vi "st_independent seeds.vi"(9 "number of seeds":i32=2, 10 "seed":i32=-1) -> (2 "independent seeds":i32[](array[numeric]))   [LabVIEW 2014, in "NI_Gmath.lvlib"]
uses:
  NI_Gmath.lvlib
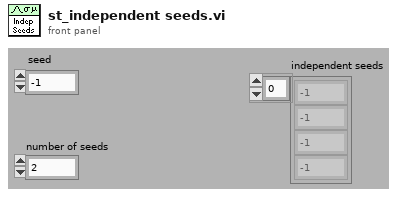
[diagram p1: front panel]
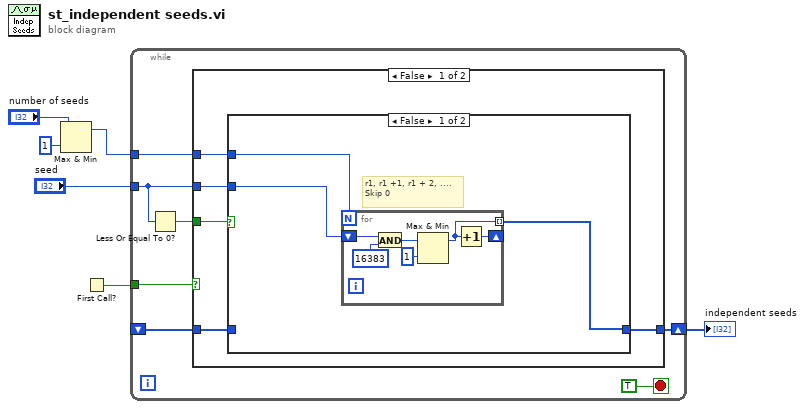
[diagram p0: block diagram]
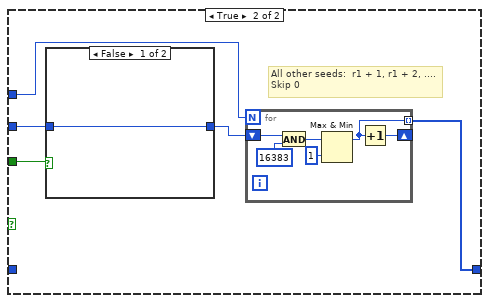
[diagram p3: hidden frame]
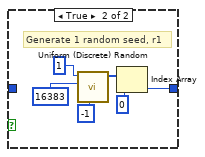
[diagram p4: hidden frame]
diagram:
  n1 = Max & Min(x="number of seeds", y=1) -> (max(x,y)=w2:i32)  [unwired: 1 out]
  n2 = First Call?() -> (First Call?: T/F=w5:bool)
  n3 = while {
    tunnel: w2 -> [w13]
    tunnel: "seed" -> [w11]
    shift-right: [w7] -> w1
    shift-left: _ -> [w12]
    tunnel: w5 -> [w9]
    stop <- TRUE stop-if-true
    n4 = Less Or Equal To 0?(x=w11) -> (x <= 0?=w10:bool)
    n5 = case shown="False" w9 {
      tunnel: w13 -> [w14 w31]
      tunnel: w11 -> [w15 w33]
      tunnel: w12 -> [w17 _]
      tunnel: w10 -> [w18 w32]
      tunnel: [w16 w30] -> w7
      frame False {
        n6 = case shown="False" w18 {
          tunnel: w17 -> [_ w28]
          tunnel: [w19 w28] -> w16
          tunnel: w15 -> [w21 _]
          tunnel: w14 -> [w20 _]
          frame False {
            # "r1, r1 +1, r1 + 2, ....\nSkip 0"
            n7 = for {
              N: w20 -> [_]
              shift-right: [w24] -> _
              shift-left: w21 -> [w23]
              tunnel: [w22] -> w19 mode=indexing
              n8 = And(x=w23, y=16383 ("x")) -> (x .and. y?=w25:i32)
              n9 = Max & Min(x=w25, y=1) -> (max(x,y)=w22:i32)  [unwired: 1 out]
              n10 = Increment(x=w22) -> (x+1=w24:i32)
            }
          }
          frame True {
          }
        }
      }
      frame True {
        # "All other seeds:  r1 + 1, r1 + 2, ....\nSkip 0"
        n11 = case shown="False" w32 {
          tunnel: w33 -> [w40 _]
          tunnel: [w40 w41] -> w29
          frame False {
          }
          frame True {
            # "Generate 1 random seed, r1"
            n12 = call "Uniform (Discrete) Random.vi"("seed"=-1, "n"=16383 ("x"), "samples"=1) -> ("uniform (discrete) random data"=w43:i32[])  [unwired: 7 in, 1 out]
            n13 = Index Array(array=w43, index=0) -> (element=w41:i32)
          }
        }
        n14 = for {
          N: w31 -> [_]
          shift-right: [w36] -> _
          shift-left: w29 -> [w35]
          tunnel: [w34] -> w30 mode=indexing
          n15 = And(x=w35, y=16383 ("x")) -> (x .and. y?=w37:i32)
          n16 = Max & Min(x=w37, y=1) -> (max(x,y)=w34:i32)  [unwired: 1 out]
          n17 = Increment(x=w34) -> (x+1=w36:i32)
        }
      }
    }
  }
  "independent seeds" <- w1
